vi "CalcTheta.vi"() -> (3 "ThetaValues":dbl[](array[numeric]))   [LabVIEW 2018]
panel:
  in  "W":dbl=23.375
  in  "L":dbl=21.5
  # "Input length/width:"
  # "Front of bot"
  # "L"
  # "W"
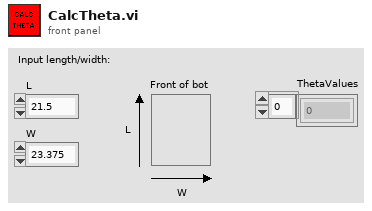
[diagram p1: front panel]
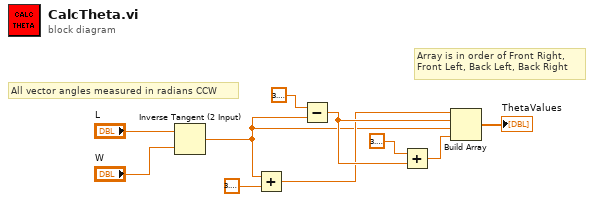
[diagram p0: block diagram]
diagram:
  # "Array is in order of Front Right,\nFront Left, Back Left, Back Right"
  # "All vector angles measured in radians CCW"
  n1 = Inverse Tangent (2 Input)(1:"W", 2:"L") -> (0:w1:dbl)
  n2 = Add(x=w1, y=3.141592653589793) -> (x+y=w2:dbl)
  n3 = Subtract(x=3.141592653589793, y=w1) -> (x-y=w3:dbl)
  n4 = Add(x=3.141592653589793, y=w3) -> (x+y=w4:dbl)
  n5 = Build Array(w2, w3, w1, w4) -> (→"ThetaValues":dbl[])
